vi "Save Short Help.vi"(8 "error in (no error)":errorcluster, 10 "path":path, 11 "vi ref":refnum<vi>) -> (0 "error out":errorcluster, 2 "path out":path, 3 "reference out":refnum<vi>)   [LabVIEW 2014, in "lvprj2html.lvlib"]
uses:
  lvprj2html.lvlib
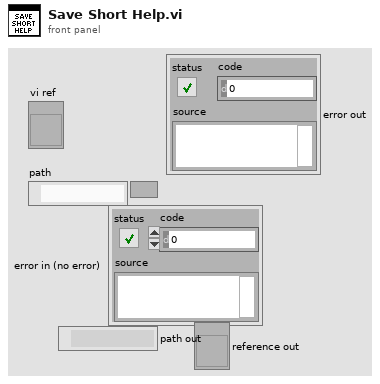
[diagram p1: front panel]
types:
  T1 = enum32{"Custom", "Standard", "Using Panel", "Using SubVI", "Complete"}
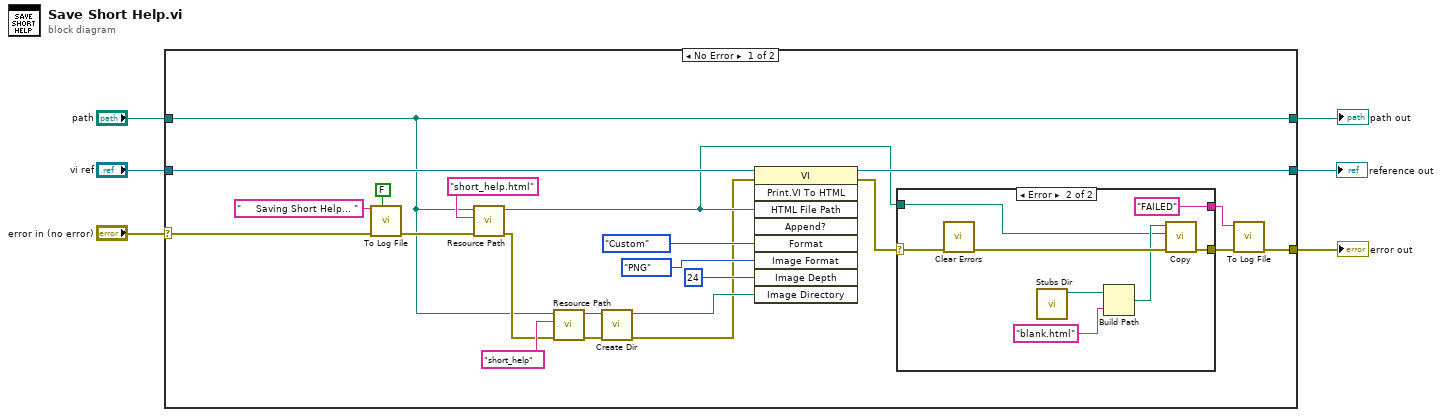
[diagram p0: block diagram]
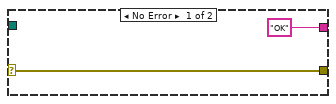
[diagram p2: hidden frame]
diagram:
  n1 = case shown="No Error" "error in (no error)" {
    selector: "error in (no error)" -> [w17 w39]
    tunnel: "vi ref" -> [w28 w40]
    tunnel: "path" -> [w16 w41]
    tunnel: [w21 w40] -> w4
    tunnel: [w11 w39] -> w3
    tunnel: [w16 w41] -> w1
    frame No Error {
      n2 = call "To Log File.vi"("new line"=FALSE, "error in (no error)"=w17, "string"="     Saving Short Help... " ("format string")) -> ("error out"=w18:errorcluster)  [unwired: 8 in]
      n3 = call "Resource Path.vi"("error in (no error)"=w18, "resource file name"="short_help.html", "data dir"=w16) -> ("error out"=w22:errorcluster, "path"=w12:path)  [unwired: 7 in]
      n4 = call "Resource Path.vi"("error in (no error)"=w22, "resource file name"="short_help", "data dir"=w16) -> ("error out"=w9:errorcluster, "path"=w10:path)  [unwired: 7 in]
      n5 = call "Create Dir.vi"("error in (no error)"=w9, "appended path"=w10) -> ("error out"=w7:errorcluster, "created path"=w8:path)  [unwired: 8 in]
      n6 = invoke class="VI" method="Print.VI To HTML"(reference=w28, error in=w7, "HTML File Path"=w12, "Format"=T1."Custom", "Image Format"=enum32{"PNG", "JPEG", "GIF"}."PNG", "Image Depth"=24, "Image Directory"=w8) -> (reference out=w21:refnum<vi>, error out=w13:errorcluster)  [unwired: 2 in, 7 out]
      n7 = case shown="Error" w13 {
        selector: w13 -> [w30 w38]
        tunnel: [w30 w32] -> w15
        tunnel: ["OK" ("string") "FAILED" ("string")] -> w14
        tunnel: w12 -> [_ w33]
        frame No Error {
        }
        frame Error {
          n8 = call <vilib>:"Clear Errors.vi"("error in (no error)"=w38) -> ("error out"=w35:errorcluster)  [unwired: 5 in, 1 out]
          n9 = call "Stubs Dir.vi"() -> ("path"=w31:path)  [unwired: 11 in]
          n10 = Build Path(base path=w31, name or relative path="blank.html") -> (appended path=w34:path)
          n11 = call "Copy.vi"("error in (no error)"=w35, "dst"=w33, "src"=w34) -> ("error out"=w32:errorcluster)  [unwired: 8 in]
        }
      }
      n12 = call "To Log File.vi"("error in (no error)"=w15, "string"=w14) -> ("error out"=w11:errorcluster)  [unwired: 9 in]
    }
    frame Error {
    }
  }
  "error out" <- w3
  "reference out" <- w4
  "path out" <- w1
